vi "TCP_client.vi"(8 "error in (no error)":errorcluster, 10 "data_q":refnum<queue>, 11 "client":refnum<queue>) -> (0 "error out":errorcluster)   [LabVIEW 2023]
uses:
  tcp_enum.ctl
  Labview/img_data.ctl
  <vilib>/picture/picture.llb/imagedata.ctl
  Labview/data_commands.ctl
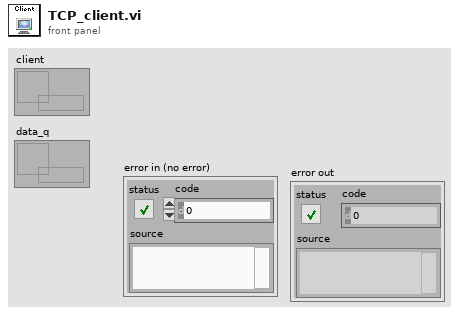
[diagram p1: front panel]
types:
  T1 = typedef "data_commands.ctl" = enum16{"stop", "bin", "edg", "gauss", "blurr", "idle"}
  T2 = typedef "tcp_enum.ctl" = enum16{"idle", "stop", "connect"}
  T3 = typedef "img_data.ctl" = cluster{"ori":T4, "curent":T4, "comands":T1}
  T4 = typedef "imagedata.ctl" = cluster{"image type":i32, "image depth":i32, "image":u8[], "mask":u8[], "colors":u32[], "Rectangle":cluster{"left":i16, "top":i16, "right":i16, "bottom":i16}}
  T5 = enum16{"Standard", "Buffered", "CRLF", "Immediate"}
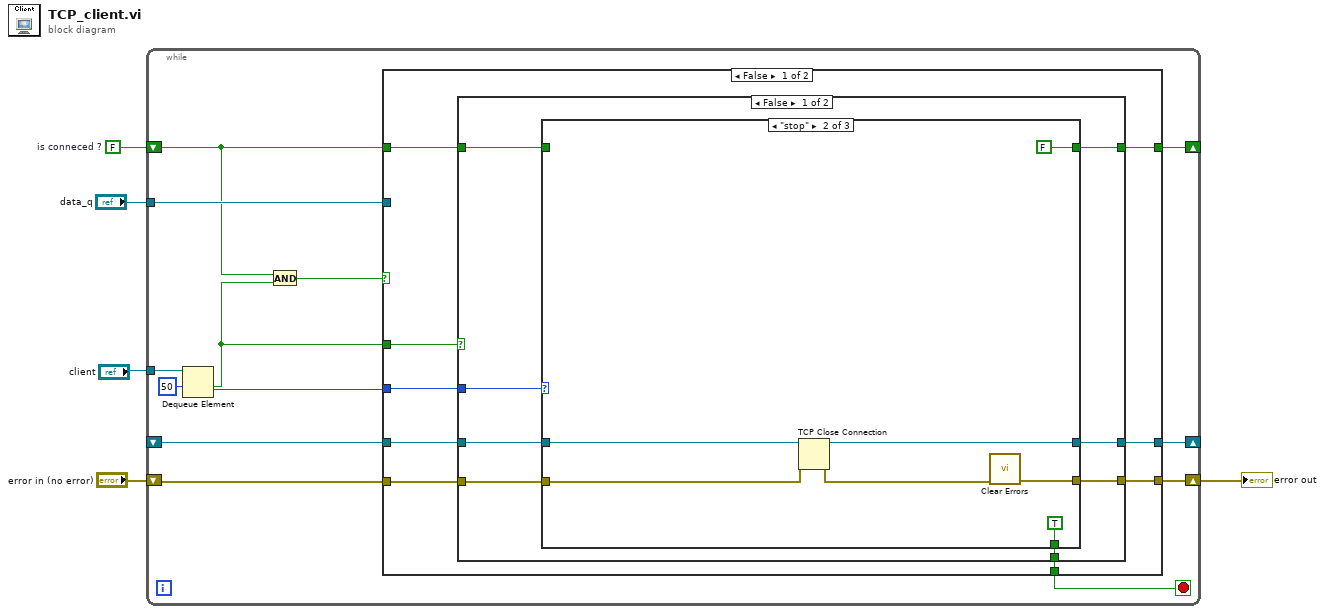
[diagram p0: block diagram]
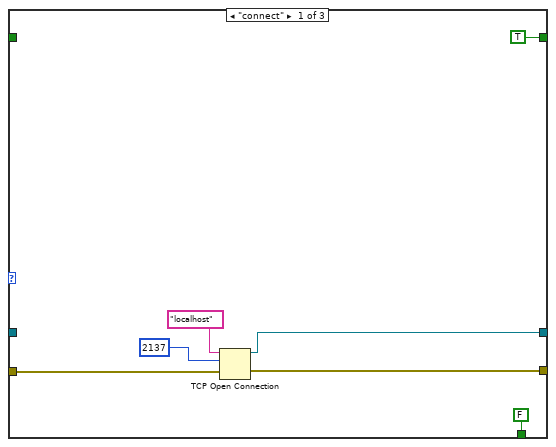
[diagram p2: hidden frame]
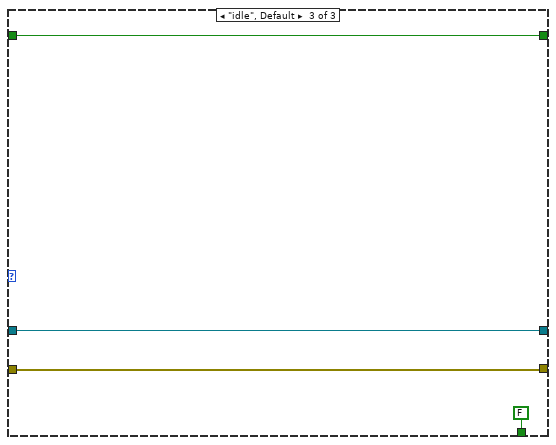
[diagram p3: hidden frame]
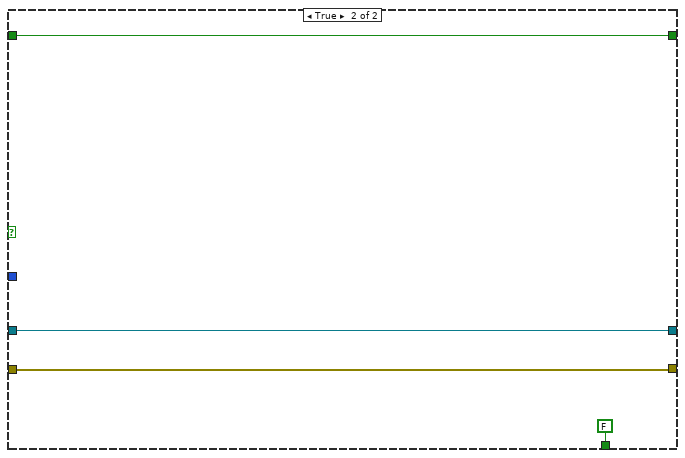
[diagram p4: hidden frame]
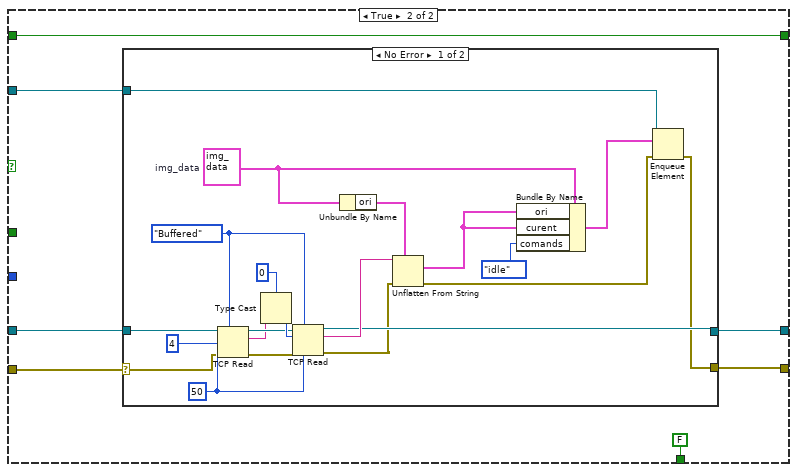
[diagram p5: hidden frame]
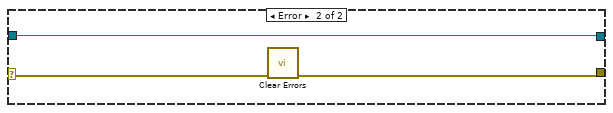
[diagram p6: hidden frame]
diagram:
  w1 = FALSE  # is conneced ?
  n1 = while {
    shift-right: [w10] -> w4
    shift-left: "error in (no error)" -> [w15]
    tunnel: "client" -> [w18]
    shift-right: [w9] -> _
    shift-left: _ -> [w14]
    tunnel: "data_q" -> [w16]
    shift-right: [w8] -> _
    shift-left: w1 -> [w13]
    stop <- w7 stop-if-true
    n2 = Dequeue Element(queue=w18, timeout in ms (-1)=50) -> (element=w11:T2, timed out?=w12:bool)  [unwired: 1 in, 2 out]
    n3 = And(x=w13, y=w12) -> (x .and. y?=w17:bool)
    n4 = case shown="False" w17 {
      tunnel: w16 -> [_ w63]
      tunnel: w15 -> [w25 w62]
      tunnel: w14 -> [w20 w61]
      tunnel: w13 -> [w21 w64]
      tunnel: w12 -> [w27 _]
      tunnel: w11 -> [w26 _]
      tunnel: [w24 w59] -> w10
      tunnel: [w23 w60] -> w9
      tunnel: [w22 w64] -> w8
      tunnel: [w19 FALSE] -> w7
      frame False {
        n5 = case shown="False" w27 {
          tunnel: w26 -> [w35 _]
          tunnel: w25 -> [w34 w55]
          tunnel: [w33 w55] -> w24
          tunnel: [w32 w56] -> w23
          tunnel: [w31 w57] -> w22
          tunnel: w21 -> [w28 w57]
          tunnel: w20 -> [w29 w56]
          tunnel: [w30 FALSE] -> w19
          frame False {
            n6 = case shown="\"stop\"" w35 {
              tunnel: w34 -> [w42 w45 w52]
              tunnel: [w41 w43 w52] -> w33
              tunnel: [w40 w46 w53] -> w32
              tunnel: [TRUE FALSE w51] -> w31
              tunnel: [FALSE TRUE FALSE] -> w30
              tunnel: w29 -> [_ w47 w53]
              tunnel: w28 -> [_ _ w51]
              frame "connect" {
                n7 = TCP Open Connection(address="localhost", remote port or service name=u16 2137, error in (no error)=w42) -> (connection ID=w40:refnum<k5>, error out=w41:errorcluster)  [unwired: 2 in]
              }
              frame "stop" {
                n8 = TCP Close Connection(connection ID=w47, error in (no error)=w45) -> (connection ID out=w46:refnum<k5>, error out=w44:errorcluster)  [unwired: 1 in]
                n9 = call <vilib>:"Clear Errors.vi"("error in (no error)"=w44) -> ("error out"=w43:errorcluster)  [unwired: 5 in, 1 out]
              }
              frame "idle", Default {
              }
            }
          }
          frame True {
          }
        }
      }
      frame True {
        n10 = case shown="No Error" w62 {
          selector: w62 -> [w69 w86]
          tunnel: w61 -> [w78 w87]
          tunnel: [w65 w88] -> w59
          tunnel: [w81 w87] -> w60
          tunnel: w63 -> [w74 _]
          frame No Error {
            w70 = T3 {"ori"={"image type"=0, "image depth"=0, "image"=[], "mask"=[], "colors"=[], "Rectangle"={"left"=0, "top"=0, "right"=0, "bottom"=0}}, "curent"={"image type"=0, "image depth"=0, "image"=[], "mask"=[], "colors"=[], "Rectangle"={"left"=0, "top"=0, "right"=0, "bottom"=0}}, "comands"=enum."bin"}  # img_data
            w76 = T5."Buffered" ("mode (standard)")
            w75 = 50 ("timeout ms (25000)")
            n11 = TCP Read(connection ID=w78, bytes to read=4, error in (no error)=w69, 7:w76, 9:w75) -> (connection ID out=w80:refnum<k5>, data out=w71:string, error out=w77:errorcluster)
            n12 = Type Cast(type=u32 0, x=w71) -> (*(type *) &x=w82:u32)
            n13 = TCP Read(connection ID=w80, bytes to read=w82, error in (no error)=w77, 7:w76, 9:w75) -> (connection ID out=w81:refnum<k5>, data out=w83:string, error out=w67:errorcluster)
            n14 = Unbundle By Name(w70) -> ("ori"=w84:T4)
            n15 = Unflatten From String(type=w84, binary string=w83, error in (no error)=w67) -> (value=w85:T4, error out=w66:errorcluster)  [unwired: 2 in, 1 out]
            n16 = Bundle By Name(cluster=w70, "ori"=w85, "curent"=w85, "comands"=data_commands."idle") -> (w73:T3)
            n17 = Enqueue Element(queue=w74, element=w73, error in (no error)=w66) -> (error out=w65:errorcluster)  [unwired: 1 in, 2 out]
          }
          frame Error {
            n18 = call <vilib>:"Clear Errors.vi"("error in (no error)"=w86) -> ("error out"=w88:errorcluster)  [unwired: 5 in, 1 out]
          }
        }
      }
    }
  }
  "error out" <- w4
